vi "CloseBaxterCamera.vi"(0 "error in":errorcluster, 2 "Camera":T1, 3 "node":string) -> (1 "error out":errorcluster)   [LabVIEW 2016]
doc: "Closes the connection to a camera"
uses:
  ROS/Code/SubVIs/BaxterCamera.ctl
  ROS/Code/Console/Servers/ServerSubs/TopicDef.ctl
  ROS/Code/SubVIs/_ROSDirection.ctl
  ROS/MessageBuilding/std_msgs/subs/stringScalar.vi
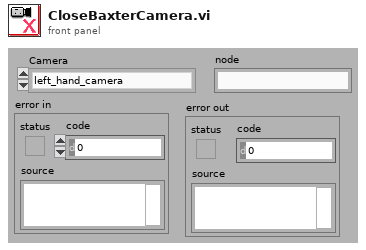
[diagram p1: front panel]
types:
  T1 = typedef "BaxterCamera.ctl" = enum16{"left_hand_camera", "right_hand_camera", "head_camera"}
  T2 = typedef "TopicDef.ctl" = cluster{"Topic":string, "Type":string, "Action":T3, "Update (ms)":u16, "queue size":u16}
  T3 = typedef "_ROSDirection.ctl" = enum16{"Node", "Publisher", "Subscriber", "ServiceClient", "ServiceProvider"}
  T4 = typedef "_ROSControl.ctl" = cluster{"topic port":u16, "Node":string, "topic":string, "type":string, "node port":u16, "error ":errorcluster, "Direction":T3, "Update (ms)":u16, "FIFO size":u16}
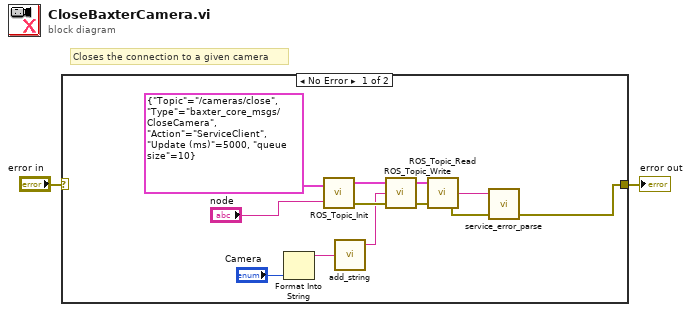
[diagram p0: block diagram]
diagram:
  # "Closes the connection to a given camera"
  n1 = case shown="No Error" "error in" {
    selector: "error in" -> [_ w15]
    tunnel: [w3 w15] -> w2
    frame No Error {
      n2 = Format Into String("Camera") -> (resulting string=w9:string)  [unwired: 3 in, 1 out]
      n3 = call "ROS_Topic_Init.vi"("Definitions"=T2 {"Topic"="/cameras/close", "Type"="baxter_core_msgs/CloseCamera", "Action"=enum."ServiceClient", "Update (ms)"=5000, "queue size"=10}, "node"="node") -> ("ROS out"=w13:T4, "error out"=w7:errorcluster)  [unwired: 1 in]
      n4 = call-poly "add_string.vi"("String"=w9) -> ("msg out"=w5:string)  [unwired: 4 in]
      n5 = call "ROS_Topic_Write.vi"("error in (no error)"=w7, "Msg in"=w5, "ROS in"=w13) -> ("error out"=w6:errorcluster, "ROS out"=w12:T4)  [unwired: 1 in]
      n6 = call "ROS_Topic_Read.vi"("error in (no error)"=w6, "ROS in"=w12) -> ("error out"=w4:errorcluster, "Reply"=w11:string)  [unwired: 1 in, 1 out]
      n7 = call "service_error_parse.vi"("error in (no error)"=w4, "Reply"=w11) -> ("error out"=w3:errorcluster)  [unwired: 1 in, 2 out]
    }
    frame Error {
    }
  }
  "error out" <- w2
